vi "Finish.vi"   [LabVIEW 2012]
doc: "This VI is called just before exiting. It is expected to close I/O refnum, save collected data, etc."
uses:
  <vilib>/Rock Robotics/WPI/Compressor/WPI_CompressorGetSetRefNum.vi
  <vilib>/Rock Robotics/WPI/Joystick/WPI_JoystickGetSetRefNum.vi
  <vilib>/Rock Robotics/WPI/RobotDrive/WPI_RobotDriveGetSetRefNum.vi
types:
  T1 = typedef "WPI_MotorControlDeviceRef.ctl" = cluster{"DeviceStatus":errorcluster, "Type":enum16{"PWM", "CAN"}, "PWM":cluster{"Digital Module":T2, "PWM Channel":T3, "DeadBand":T4}, "CAN":cluster{"Device Number":u8, "Control Mode":T5, "Semaphore":T6, "Max Vout":dbl}, "Invert":bool, "TransformRef":T7, "InvTransformRef":T7}
  T2 = typedef "FPGA_TypedefDigitalModule.ctl" = enum16{"Digital Module 1", "Digital Module 2"}
  T3 = typedef "FPGA_DIOPWMChannel.ctl" = enum8{"PWM 1", "PWM 2", "PWM 3", "PWM 4", "PWM 5", "PWM 6", "PWM 7", "PWM 8", "PWM 9", "PWM 10", "Invalid"}
  T4 = typedef "WPI_PWMDeadband.ctl" = cluster{"Name":string, "maxPositivePwm":i32, "minPositivePwm":i32, "centerPwm":i32, "maxNegativePwm":i32, "minNegativePwm":i32, "angularRange":u16}
  T5 = typedef "WPI_CANJaguar_ControlMode.ctl" = enum8{"Percent VBus", "Current", "Speed", "Position", "Voltage"}
  T6 = typedef "Semaphore RefNum" = refnum<k1>
  T7 = typedef "WPI_PWMTransform_ConPane.ctl" = refnum<vi>
  T8 = typedef "WPI_CompressorDevRef.ctl" = cluster{"DevStatus":errorcluster, "DigitalInputDevRef":T9, "RelayDevRef":T11}
  T9 = typedef "WPI_DigitalInputDevRef.ctl" = cluster{"DevStatus":errorcluster, "DIO Channel":T10, "Digital Module":T2}
  T10 = typedef "FPGA_DIOChannel.ctl" = enum8{"DIO 1", "DIO 2", "DIO 3", "DIO 4", "DIO 5", "DIO 6", "DIO 7", "DIO 8", "DIO 9", "DIO 10", "DIO 11", "DIO 12", "DIO 13", "DIO 14", "Invalid"}
  T11 = typedef "WPI_RelayDevRef.ctl" = cluster{"DevStatus":errorcluster, "Relay Channel":T12, "Digital Module":T2, "Relay Direction":T13}
  T12 = typedef "FPGA_DIORelayChannel.ctl" = enum8{"Relay 1", "Relay 2", "Relay 3", "Relay 4", "Relay 5", "Relay 6", "Relay 7", "Relay 8", "Invalid"}
  T13 = typedef "WPI_RelayDirection.ctl" = enum16{"Both directions", "Forward only", "Reverse only"}
  T14 = typedef "WPI_AnalogChannelDevRef.ctl" = cluster{"DevStatus":errorcluster, "Analog Module":T15, "Analog Channel":T16}
  T15 = typedef "FPGA_TypedefAnalogModule.ctl" = enum16{"Analog Module 1", "Analog Module 2"}
  T16 = typedef "FPGA_AIChannel.ctl" = enum8{"AI 1", "AI 2", "AI 3", "AI 4", "AI 5", "AI 6", "AI 7", "AI 8", "Invalid"}
  T17 = typedef "WPI_CounterDevRef.ctl" = cluster{"DevStatus":errorcluster, "CntIndex":T18}
  T18 = typedef "FPGA_CounterCtrSystemIndex.ctl" = enum8{"Ctr 0", "Ctr 1", "Ctr 2", "Ctr 3", "Ctr 4", "Ctr 5", "Ctr 6", "Ctr 7", "Invalid"}
  T19 = typedef "WPI_JoystickDevRef.ctl" = cluster{"Device":T20}
  T20 = typedef "WPI_JoystickDeviceEnum.ctl" = enum16{"USB 1", "USB 2", "USB 3", "USB 4", "Kinect 1", "Kinect 2"}
  T21 = typedef "WPI_RobotDriveDevRef.ctl" = cluster{"DevStatus":errorcluster, "Motors[]":T1[], "Square Inputs":bool, "Max Output":dbl, "Isochronous":bool}
  T22 = typedef "WPI_SolenoidDevRef.ctl" = cluster{"DevStatus":errorcluster, "Solenoid Module":T23, "Forward Solenoid Channel":T24, "Reverse Solenoid Channel":T24}
  T23 = typedef "FPGA_TypedefSolenoidModule.ctl" = enum16{"Solenoid Module 1", "Solenoid Module 2"}
  T24 = typedef "WPI_SolenoidChannel.ctl" = enum8{"Solenoid 1", "Solenoid 2", "Solenoid 3", "Solenoid 4", "Solenoid 5", "Solenoid 6", "Solenoid 7", "Solenoid 8", "Invalid"}
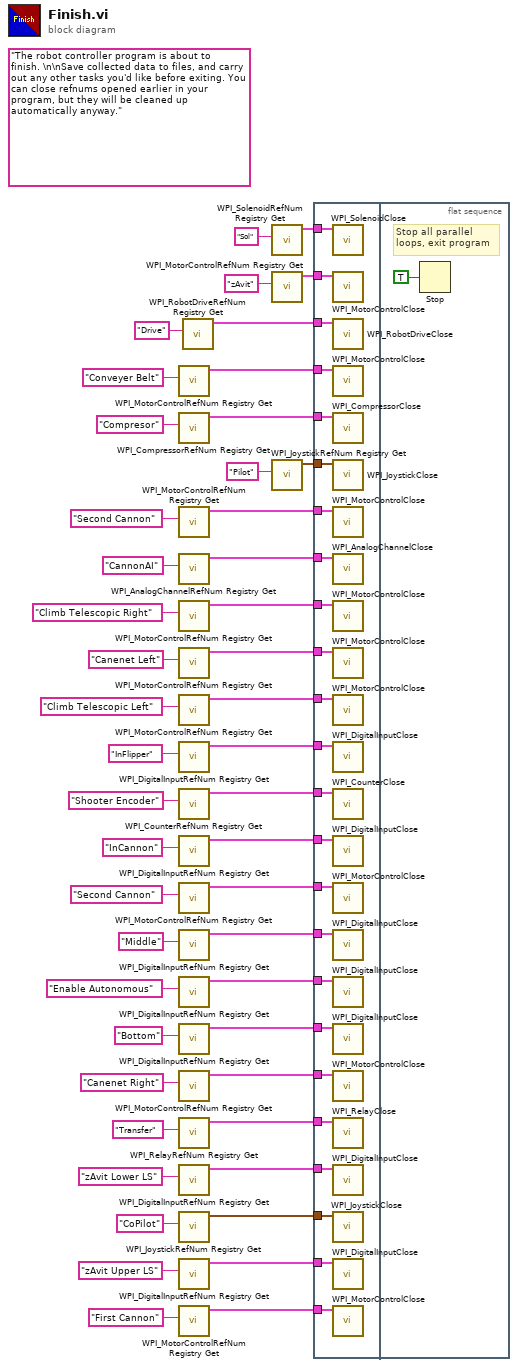
[diagram p0: block diagram]
diagram:
  (unwired) "The robot controller program is about to finish. \n\nSave collected data to files, and carry out any other tasks you'd like before exiting. You can close refnums opened earlier in your program, but they will be cleaned up automatically anyway."
  n1 = call <vilib>:"WPI_MotorControlRefNum Registry Get.vi"("refnum name"="Conveyer Belt") -> ("MotorControlDevRef"=w35:T1)  [unwired: 9 in, 1 out]
  n2 = call <vilib>:"WPI_CompressorRefNum Registry Get.vi"("refnum name"="Compresor") -> ("CompressorDevRef"=w4:T8)  [unwired: 9 in, 1 out]
  n3 = call <vilib>:"WPI_MotorControlRefNum Registry Get.vi"("refnum name"="Second Cannon") -> ("MotorControlDevRef"=w41:T1)  [unwired: 9 in, 1 out]
  n4 = call <vilib>:"WPI_AnalogChannelRefNum Registry Get.vi"("refnum name"="CannonAI") -> ("AIDeviceRef"=w9:T14)  [unwired: 9 in, 1 out]
  n5 = call <vilib>:"WPI_MotorControlRefNum Registry Get.vi"("refnum name"="Climb Telescopic Right") -> ("MotorControlDevRef"=w17:T1)  [unwired: 9 in, 1 out]
  n6 = call <vilib>:"WPI_MotorControlRefNum Registry Get.vi"("refnum name"="Canenet Left") -> ("MotorControlDevRef"=w19:T1)  [unwired: 9 in, 1 out]
  n7 = call <vilib>:"WPI_MotorControlRefNum Registry Get.vi"("refnum name"="Climb Telescopic Left") -> ("MotorControlDevRef"=w20:T1)  [unwired: 9 in, 1 out]
  n8 = call <vilib>:"WPI_DigitalInputRefNum Registry Get.vi"("refnum name"="InFlipper") -> ("DigitalInputDevRef"=w25:T9)  [unwired: 9 in, 1 out]
  n9 = call <vilib>:"WPI_CounterRefNum Registry Get.vi"("refnum name"="Shooter Encoder") -> ("CounterDevRef"=w1:T17)  [unwired: 9 in, 1 out]
  n10 = call <vilib>:"WPI_DigitalInputRefNum Registry Get.vi"("refnum name"="InCannon") -> ("DigitalInputDevRef"=w26:T9)  [unwired: 9 in, 1 out]
  n11 = call <vilib>:"WPI_MotorControlRefNum Registry Get.vi"("refnum name"="Second Cannon") -> ("MotorControlDevRef"=w7:T1)  [unwired: 9 in, 1 out]
  n12 = call <vilib>:"WPI_DigitalInputRefNum Registry Get.vi"("refnum name"="Middle") -> ("DigitalInputDevRef"=w27:T9)  [unwired: 9 in, 1 out]
  n13 = call <vilib>:"WPI_DigitalInputRefNum Registry Get.vi"("refnum name"="Enable Autonomous") -> ("DigitalInputDevRef"=w11:T9)  [unwired: 9 in, 1 out]
  n14 = call <vilib>:"WPI_DigitalInputRefNum Registry Get.vi"("refnum name"="Bottom") -> ("DigitalInputDevRef"=w28:T9)  [unwired: 9 in, 1 out]
  n15 = call <vilib>:"WPI_MotorControlRefNum Registry Get.vi"("refnum name"="Canenet Right") -> ("MotorControlDevRef"=w18:T1)  [unwired: 9 in, 1 out]
  n16 = call <vilib>:"WPI_RelayRefNum Registry Get.vi"("refnum name"="Transfer") -> ("RelayDevRef"=w33:T11)  [unwired: 9 in, 1 out]
  n17 = call <vilib>:"WPI_DigitalInputRefNum Registry Get.vi"("refnum name"="zAvit Lower LS") -> ("DigitalInputDevRef"=w13:T9)  [unwired: 9 in, 1 out]
  n18 = call <vilib>:"WPI_JoystickRefNum Registry Get.vi"("refnum name"="CoPilot") -> ("JoystickDevRef"=w38:T19)  [unwired: 9 in, 1 out]
  n19 = call <vilib>:"WPI_DigitalInputRefNum Registry Get.vi"("refnum name"="zAvit Upper LS") -> ("DigitalInputDevRef"=w14:T9)  [unwired: 9 in, 1 out]
  n20 = call <vilib>:"WPI_MotorControlRefNum Registry Get.vi"("refnum name"="First Cannon") -> ("MotorControlDevRef"=w40:T1)  [unwired: 9 in, 1 out]
  n21 = call <vilib>:"WPI_RobotDriveRefNum Registry Get.vi"("refnum name"="Drive") -> ("RobotDriveDevRef"=w48:T21)  [unwired: 1 in, 9 out]
  n22 = call <vilib>:"WPI_SolenoidRefNum Registry Get.vi"("refnum name"="Sol") -> ("SolenoidDevRef"=w3:T22)  [unwired: 9 in, 1 out]
  n23 = call <vilib>:"WPI_MotorControlRefNum Registry Get.vi"("refnum name"="zAvit") -> ("MotorControlDevRef"=w45:T1)  [unwired: 9 in, 1 out]
  n24 = call <vilib>:"WPI_JoystickRefNum Registry Get.vi"("refnum name"="Pilot") -> ("JoystickDevRef"=w47:T19)  [unwired: 1 in, 9 out]
  n25 = flat-sequence {
    tunnel: w48 -> [w72]
    tunnel: w47 -> [w71]
    tunnel: w45 -> [w70]
    tunnel: w41 -> [w69]
    tunnel: w40 -> [w68]
    tunnel: w38 -> [w67]
    tunnel: w35 -> [w66]
    tunnel: w33 -> [w65]
    tunnel: w28 -> [w64]
    tunnel: w27 -> [w63]
    tunnel: w26 -> [w62]
    tunnel: w25 -> [w61]
    tunnel: w20 -> [w60]
    tunnel: w19 -> [w59]
    tunnel: w18 -> [w58]
    tunnel: w17 -> [w57]
    tunnel: w14 -> [w56]
    tunnel: w13 -> [w55]
    tunnel: w11 -> [w54]
    tunnel: w9 -> [w53]
    tunnel: w7 -> [w52]
    tunnel: w4 -> [w51]
    tunnel: w3 -> [w50]
    tunnel: w1 -> [w49]
    frame #0 {
      n26 = call <vilib>:"WPI_SolenoidClose.vi"("SolenoidDevRef"=w50) -> ()  [unwired: 10 in, 1 out]
      n27 = call <vilib>:"WPI_MotorControlClose.vi"("MotorControlDevRef"=w70) -> ()  [unwired: 10 in, 1 out]
      n28 = call <vilib>:"WPI_RobotDriveClose.vi"("RobotDriveDevRef"=w72) -> ()  [unwired: 1 in, 10 out]
      n29 = call <vilib>:"WPI_MotorControlClose.vi"("MotorControlDevRef"=w66) -> ()  [unwired: 10 in, 1 out]
      n30 = call <vilib>:"WPI_CompressorClose.vi"("CompressorDevRef"=w51) -> ()  [unwired: 10 in, 1 out]
      n31 = call <vilib>:"WPI_JoystickClose.vi"("JoystickDevRef"=w71) -> ()  [unwired: 11 out]
      n32 = call <vilib>:"WPI_MotorControlClose.vi"("MotorControlDevRef"=w69) -> ()  [unwired: 10 in, 1 out]
      n33 = call <vilib>:"WPI_AnalogChannelClose.vi"("AIDeviceRef"=w53) -> ()  [unwired: 10 in, 1 out]
      n34 = call <vilib>:"WPI_MotorControlClose.vi"("MotorControlDevRef"=w57) -> ()  [unwired: 10 in, 1 out]
      n35 = call <vilib>:"WPI_MotorControlClose.vi"("MotorControlDevRef"=w59) -> ()  [unwired: 10 in, 1 out]
      n36 = call <vilib>:"WPI_MotorControlClose.vi"("MotorControlDevRef"=w60) -> ()  [unwired: 10 in, 1 out]
      n37 = call <vilib>:"WPI_DigitalInputClose.vi"("DigitalInputDevRef"=w61) -> ()  [unwired: 10 in, 1 out]
      n38 = call <vilib>:"WPI_CounterClose.vi"("CounterDevRef"=w49) -> ()  [unwired: 10 in, 1 out]
      n39 = call <vilib>:"WPI_DigitalInputClose.vi"("DigitalInputDevRef"=w62) -> ()  [unwired: 10 in, 1 out]
      n40 = call <vilib>:"WPI_MotorControlClose.vi"("MotorControlDevRef"=w52) -> ()  [unwired: 10 in, 1 out]
      n41 = call <vilib>:"WPI_DigitalInputClose.vi"("DigitalInputDevRef"=w63) -> ()  [unwired: 10 in, 1 out]
      n42 = call <vilib>:"WPI_DigitalInputClose.vi"("DigitalInputDevRef"=w54) -> ()  [unwired: 10 in, 1 out]
      n43 = call <vilib>:"WPI_DigitalInputClose.vi"("DigitalInputDevRef"=w64) -> ()  [unwired: 10 in, 1 out]
      n44 = call <vilib>:"WPI_MotorControlClose.vi"("MotorControlDevRef"=w58) -> ()  [unwired: 10 in, 1 out]
      n45 = call <vilib>:"WPI_RelayClose.vi"("RelayDevRef"=w65) -> ()  [unwired: 10 in, 1 out]
      n46 = call <vilib>:"WPI_DigitalInputClose.vi"("DigitalInputDevRef"=w55) -> ()  [unwired: 10 in, 1 out]
      n47 = call <vilib>:"WPI_JoystickClose.vi"("JoystickDevRef"=w67) -> ()  [unwired: 11 out]
      n48 = call <vilib>:"WPI_DigitalInputClose.vi"("DigitalInputDevRef"=w56) -> ()  [unwired: 10 in, 1 out]
      n49 = call <vilib>:"WPI_MotorControlClose.vi"("MotorControlDevRef"=w68) -> ()  [unwired: 10 in, 1 out]
    }
    frame #1 {
      # "Stop all parallel\nloops, exit program"
      n50 = Stop(stop? (T)=TRUE ("Quit")) -> ()
    }
  }
